vi "Send_Configuration_Keithley.vi"(7 "Filename (.ini)":string="Config_Ver_1\\Keithley_params.ini", 8 "error in":errorcluster, 11 "Keithley VISA in":refnum<visa-resource-name>) -> (0 "error out":errorcluster, 1 "List Sweep Params Out":T1 {"List Sweep Steps"."Current Level (A)" min=-0.105 max=0.105 format="%.4p"; "List Sweep Steps"."Source Delay (s)" min=0.001 max=1000.0 step=0.001 format="%.3f"; "List Sweep Steps"."Voltage Limit (V)" min=0.1 max=105.0 step=0.01 format="%.2p"}, 2 "Trig Layer Params Out":T7, 3 "Keithley VISA out":refnum<visa-resource-name>, 5 "Arm Layer Params Out":T11={"Bypass Arm Layer\nInput Trigger?"=FALSE, "Input Trig Source"=enum."Immediate", "Input Trig Link Line"=enum."1", "Arm Timer Interval (s)"=0.001, "Output Trig Mode"=enum."No Trig Out", "Output Trig Link Line"=enum."1"} {"Arm Timer Interval (s)" min=0.001 max=99999.999 step=0.001 format="%.3f"})   [LabVIEW 2021]
uses:
  <instrlib>/Keithley 622x LV 2009/Configure/Trigger/Typedefs/KE622x -- Arm Layer Params.ctl
  <instrlib>/Keithley 622x LV 2009/Configure/Trigger/Low Level/Typedefs/KE622x -- Arm Source.ctl
  <instrlib>/Keithley 622x LV 2009/Configure/Trigger/Low Level/Typedefs/KE622x -- Trig Link Line.ctl
  <instrlib>/Keithley 622x LV 2009/Configure/Trigger/Low Level/Typedefs/KE622x -- Arm Timer Interval.ctl
  <instrlib>/Keithley 622x LV 2009/Configure/Trigger/Low Level/Typedefs/KE622x -- Arm Output Mode.ctl
  <instrlib>/Keithley 622x LV 2009/Configure/Trigger/Typedefs/KE622x -- Trig Layer Params.ctl
  <instrlib>/Keithley 622x LV 2009/Configure/Trigger/Low Level/Typedefs/KE622x -- Trig Source.ctl
  <instrlib>/Keithley 622x LV 2009/Configure/Trigger/Low Level/Typedefs/KE622x -- Trig Output Mode.ctl
  <instrlib>/Keithley 622x LV 2009/Configure/Source/Typedefs/KE622x -- List Sweep Params.ctl
  <instrlib>/Keithley 622x LV 2009/Configure/Source/Typedefs/KE622x -- List Sweep Steps.ctl
  <instrlib>/Keithley 622x LV 2009/Configure/Source/Typedefs/KE622x -- List Sweep Step.ctl
  <instrlib>/Keithley 622x LV 2009/Configure/Source/Typedefs/KE622x -- Current Level.ctl
  <instrlib>/Keithley 622x LV 2009/Configure/Source/Typedefs/KE622x -- Source Delay.ctl
  <instrlib>/Keithley 622x LV 2009/Configure/Source/Typedefs/KE622x -- Voltage Limit.ctl
  <instrlib>/Keithley 622x LV 2009/Keithley 622x.lvlib
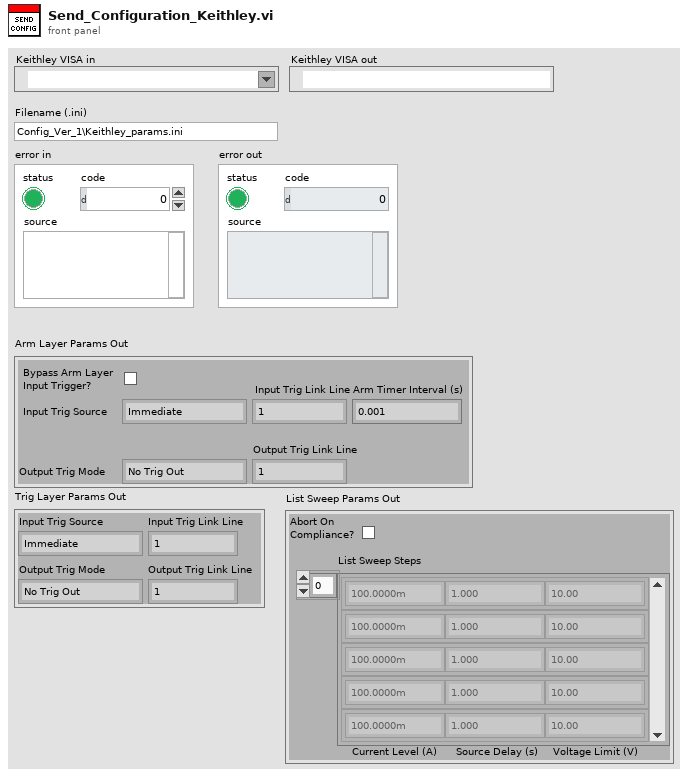
[diagram p1: front panel]
types:
  T1 = typedef "Keithley 622x.lvlib/KE622x -- List Sweep Params.ctl" = cluster{"Abort On\nCompliance?":bool, "List Sweep Steps":T2}
  T2 = typedef "Keithley 622x.lvlib/KE622x -- List Sweep Steps.ctl" = T3[]
  T3 = typedef "Keithley 622x.lvlib/KE622x -- List Sweep Step.ctl" = cluster{"Current Level (A)":T4, "Source Delay (s)":T5, "Voltage Limit (V)":T6}
  T4 = typedef "Keithley 622x.lvlib/KE622x -- Current Level.ctl" = dbl
  T5 = typedef "Keithley 622x.lvlib/KE622x -- Source Delay.ctl" = dbl
  T6 = typedef "Keithley 622x.lvlib/KE622x -- Voltage Limit.ctl" = dbl
  T7 = typedef "Keithley 622x.lvlib/KE622x -- Trig Layer Params.ctl" = cluster{"Input Trig Source":T8, "Input Trig Link Line":T9, "Output Trig Mode":T10, "Output Trig Link Line":T9}
  T8 = typedef "Keithley 622x.lvlib/KE622x -- Trig Source.ctl" = enum16{"Immediate", "Trigger Link"}
  T9 = typedef "Keithley 622x.lvlib/KE622x -- Trig Link Line.ctl" = enum16{"1", "2", "3", "4", "5", "6"}
  T10 = typedef "Keithley 622x.lvlib/KE622x -- Trig Output Mode.ctl" = enum16{"No Trig Out", "Source Turn On", "After Source Delay"}
  T11 = typedef "Keithley 622x.lvlib/KE622x -- Arm Layer Params.ctl" = cluster{"Bypass Arm Layer\nInput Trigger?":bool, "Input Trig Source":T12, "Input Trig Link Line":T9, "Arm Timer Interval (s)":T13, "Output Trig Mode":T14, "Output Trig Link Line":T9}
  T12 = typedef "Keithley 622x.lvlib/KE622x -- Arm Source.ctl" = enum16{"Immediate", "Bus (*TRG)", "Timer", "Manual", "Trigger Link", "SOT Falling Edge", "SOT Rising Edge", "SOT Either Edge"}
  T13 = typedef "Keithley 622x.lvlib/KE622x -- Arm Timer Interval.ctl" = dbl
  T14 = typedef "Keithley 622x.lvlib/KE622x -- Arm Output Mode.ctl" = enum16{"No Trig Out", "Trig Out On Enter Arm", "Trig Out On Exit Arm"}
  T15 = typedef "Keithley 622x.lvlib/KE622x -- Display Params.ctl" = cluster{"Display\nEnabled?":bool, "Custom Top\nLine Text?":bool, "Top Line Text (20 chars max)":string, "Custom Bottom\nLine Text?":bool, "Bottom Line Text (32 chars max)":string}
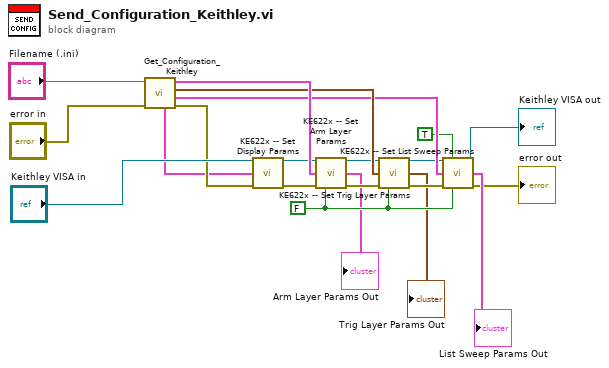
[diagram p0: block diagram]
diagram:
  w7 = FALSE ("Read Back Set Values? (T)")
  n1 = call "Get_Configuration_Keithley.vi"("error in"="error in", "Filename (.ini)"="Filename (.ini)") -> ("error out"=w18:errorcluster, "List Sweep Params In"=w14:T1, "Trig Layer Params In"=w15:T7, "Arm Layer Params In"=w16:T11, "Display Params"=w17:T15)  [unwired: 5 in]
  n2 = call <instrlib>:"KE622x -- Set Display Params.vi"("Resource In"="Keithley VISA in", "Display Params"=w17, "error in (no error)"=w18) -> ("Resource Out (dupl)"=w13:refnum<visa-resource-name>, "error out"=w12:errorcluster)  [unwired: 11 in]
  n3 = call <instrlib>:"KE622x -- Set Arm Layer Params.vi"("Resource In"=w13, "Arm Layer Params In"=w16, "error in (no error)"=w12, "Read Back Set Values? (T)"=w7) -> ("Resource Out (dupl)"=w11:refnum<visa-resource-name>, "Arm Layer Params Out"=→"Arm Layer Params Out":T11, "error out"=w10:errorcluster)  [unwired: 9 in]
  n4 = call <instrlib>:"KE622x -- Set Trig Layer Params.vi"("Resource In"=w11, "Trig Layer Params In"=w15, "error in (no error)"=w10, "Read Back Set Values? (T)"=w7) -> ("Resource Out (dupl)"=w8:refnum<visa-resource-name>, "Trig Layer Params Out"=→"Trig Layer Params Out":T7, "error out"=w9:errorcluster)  [unwired: 9 in]
  n5 = call <instrlib>:"KE622x -- Set List Sweep Params.vi"("Resource In"=w8, "Check For SCPI Errors? (T)"=TRUE, "List Sweep Params In"=w14, "error in (no error)"=w9, "Read Back Set Values? (T)"=w7) -> ("Resource Out (dupl)"=→"Keithley VISA out":refnum<visa-resource-name>, "List Sweep Params Out"=→"List Sweep Params Out":T1, "error out"=→"error out":errorcluster)  [unwired: 8 in]
